vi "main_final.vi"() -> ()   [LabVIEW 2020]
uses:
  state.ctl
  <vilib>/MakerHub/LINX/Public/Utilities/Open Serial.vi
  <vilib>/MakerHub/LINX/Public/Sensors/Motion/Servo/Servo Open One Channel.vi
  <vilib>/MakerHub/LINX/Public/Sensors/Motion/Servo/Servo Close One Channel.vi
  <vilib>/MakerHub/LINX/LMH-LINX.lvlib
  <vilib>/MakerHub/LINX/Public/Sensors/Motion/Servo/Servo.lvlib
panel:
  in  "Buzzer":u8=12
  in  "Servo":u8=11
  in  "Serial Port":refnum<visa-resource-name>="N/A"
  out "message":string
  out "temp 2":dbl format="%#_3g"
  in  "temp":dbl(slide)=23.33965844402277 scale=0.0..100.0 scale format="%#_3g"
  out "Meter":dbl(knob) scale=1.0..5.0
  out "down":bool
  out "up":bool
  out "count":i32
  in  "hold":bool
  out "5":u16(ring)
  out "4":u16(ring)
  out "3":u16(ring)
  out "2":u16(ring)
  out "1":u16(ring)
  out "1":i8
  out "2":i8
  out "4":i8
  out "3":i8
  out "5":i8
  in  "up/down":T1
  in  "floor cluster":T2
  in  "Stop":bool
  out "floor":dbl(slide) scale=10.0..50.0
  # "Reset in :"
  # "Sec"
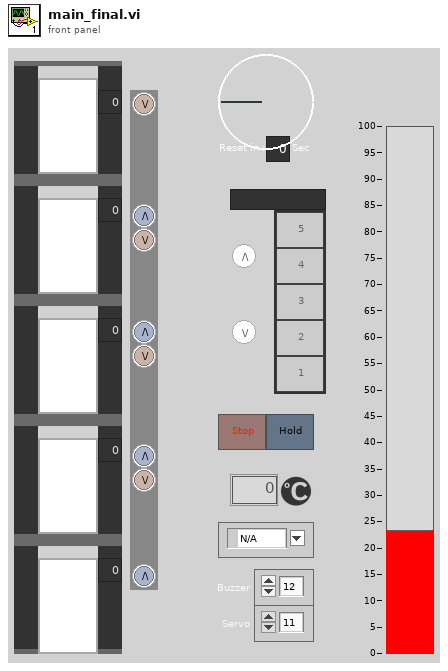
[diagram p1: front panel]
types:
  T1 = cluster{"up":bool, "down 2":bool, "up 2":bool, "down 3":bool, "up 3":bool, "down 4":bool, "up 4":bool, "down 5":bool}
  T2 = cluster{"1":bool, "2":bool, "3":bool, "4":bool, "5":bool}
  T3 = typedef "state.ctl" = enum16{"enter", "checking", "go up", "go down", "process", "get out", "temp"}
  T4 = typedef "LMH-LINX.lvlib/LINX Ref.ctl" = cluster{"IO":T5, "Interface":T6, "LINX Device Config":T7}
  T5 = typedef "LMH-LINX.lvlib/Platform.ctl" = enum16{"Remote", "Local"}
  T6 = typedef "LMH-LINX.lvlib/Interface.ctl" = enum16{"Serial", "TCP"}
  T7 = typedef "LMH-LINX.lvlib/Device.lvlib/LINX Device Config.ctl" = cluster{"Interface":T6, "COM Port":refnum<visa-resource-name>, "TCP Configuration":T8, "Device Family":u8, "Device ID":u8, "Device Name":string, "TCP Ref":refnum<k5>, "Channels":T9}
  T8 = typedef "LMH-LINX.lvlib/Device.lvlib/TCP Config.ctl" = cluster{"IP Address":string, "Port":u16}
  T9 = typedef "LMH-LINX.lvlib/Channels.ctl" = cluster{"DI":u8[], "DO":u8[], "AI":u8[], "AO":u8[], "PWM":u8[], "QE":u8[], "UART":u8[], "I2C 2":u8[], "SPI":u8[], "CAN":u8[], "Servo":u8[], "AI Ref (V)":dbl, "AI Resolution (Bits)":u8, "AO Ref (V)":dbl, "AO Resolution (Bits)":u8}
  T10 = enum8{"Enabled", "Disabled", "Disabled and Grayed Out"}
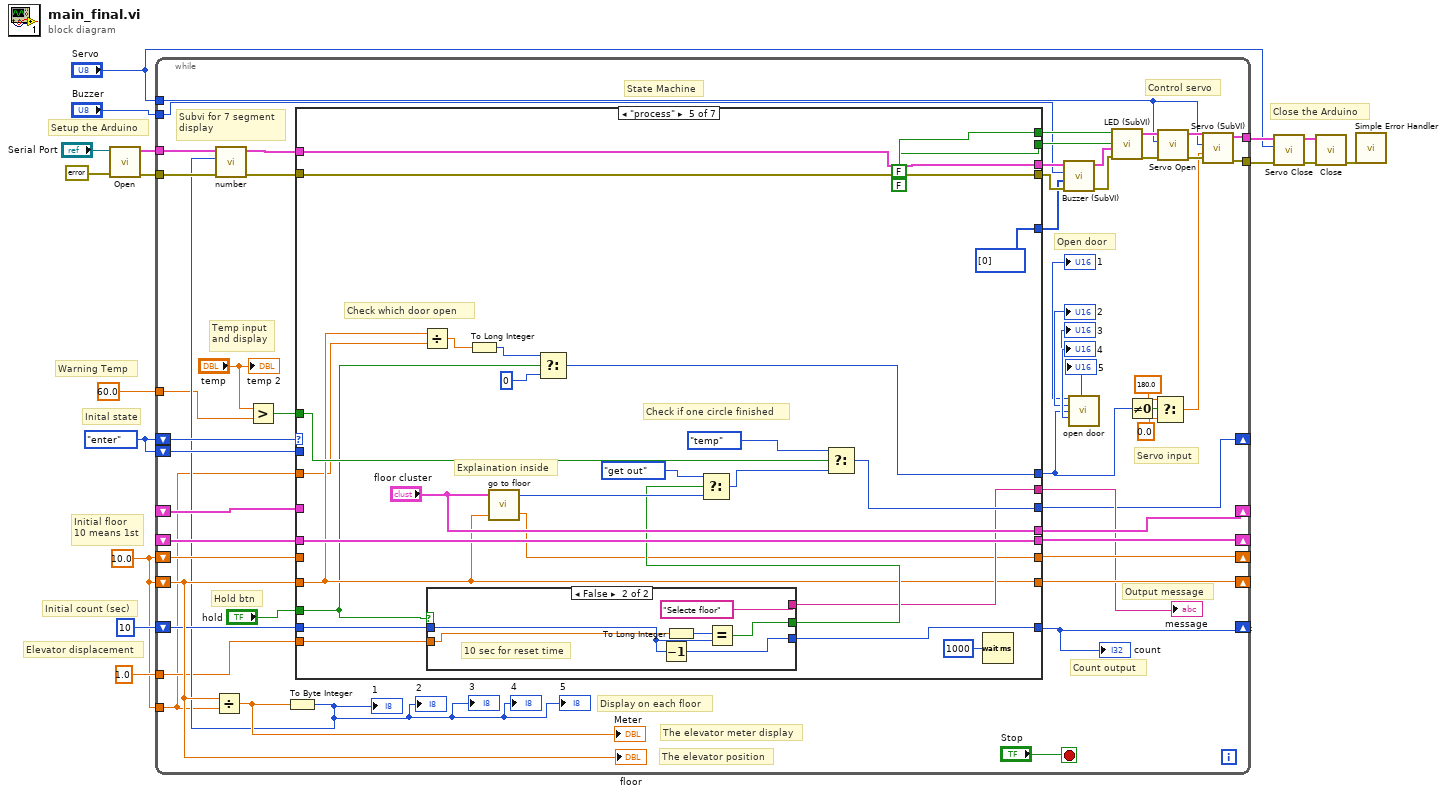
[diagram p0: block diagram]
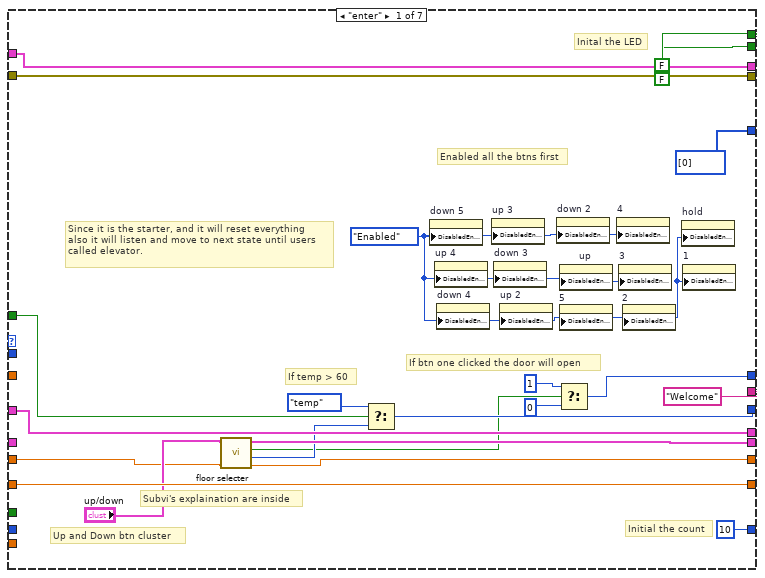
[diagram p2: hidden frame]
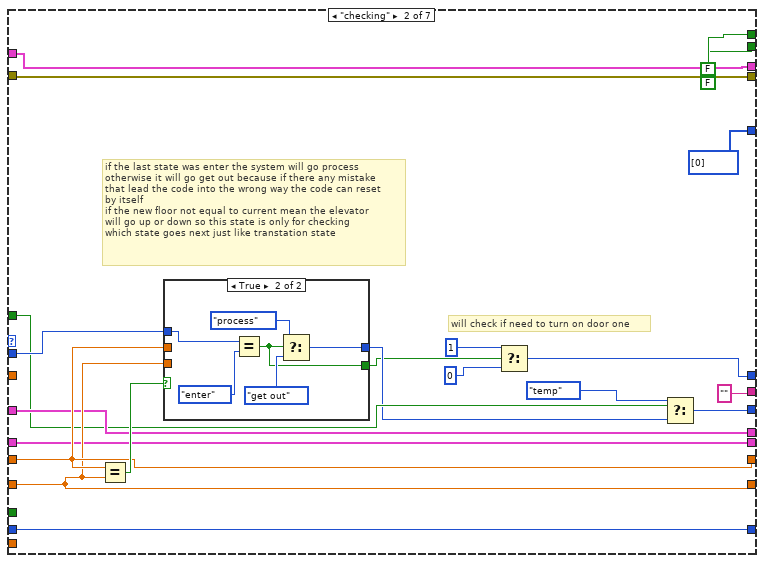
[diagram p3: hidden frame]
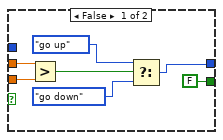
[diagram p4: hidden frame]
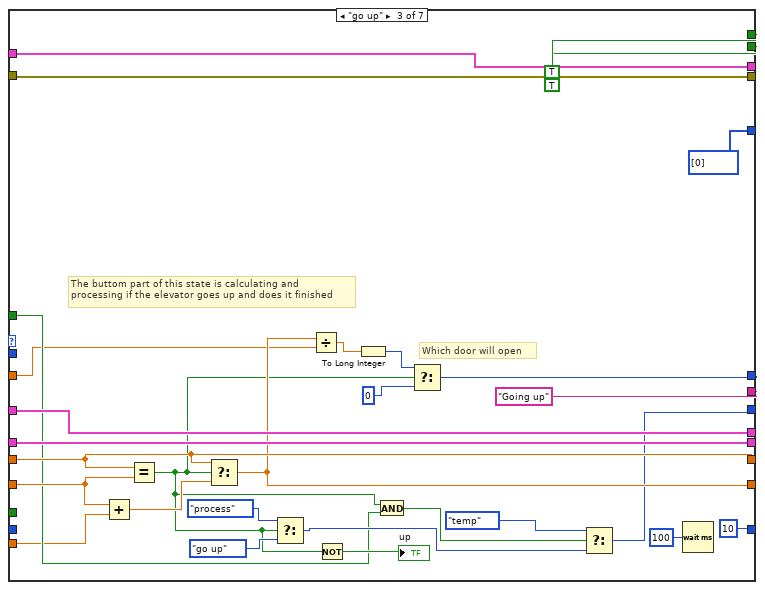
[diagram p5: hidden frame]
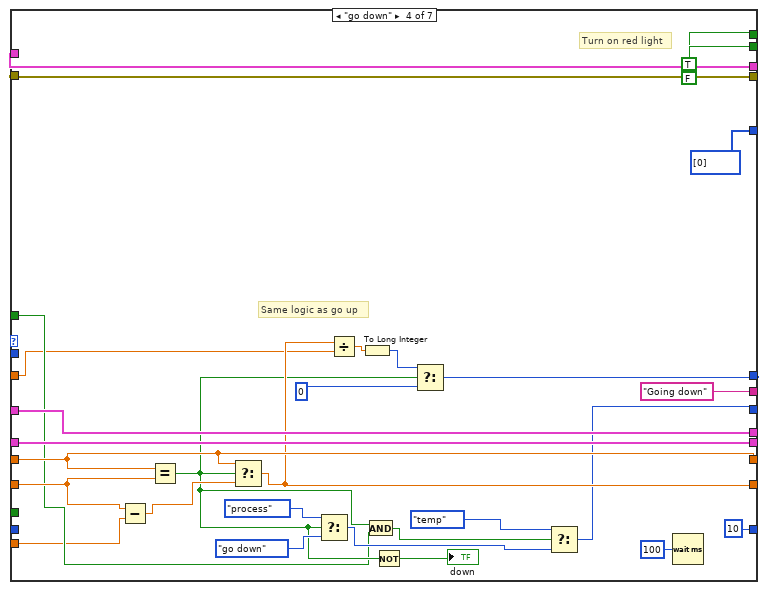
[diagram p6: hidden frame]
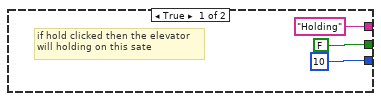
[diagram p7: hidden frame]
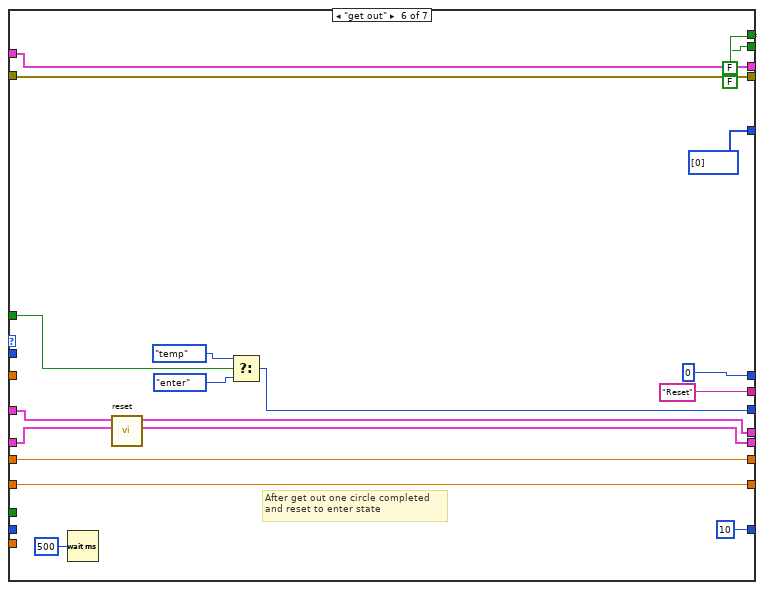
[diagram p8: hidden frame]
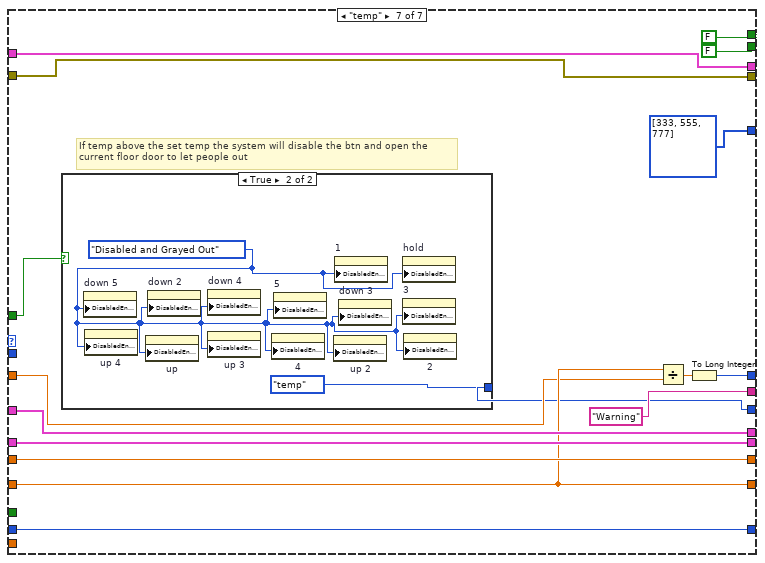
[diagram p9: hidden frame]
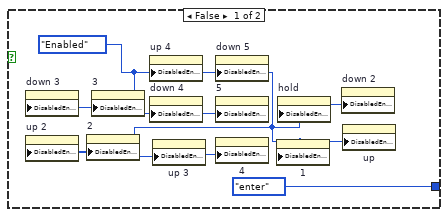
[diagram p10: hidden frame]
diagram:
  w3 = 10.0 ("floor")
  w15 = state."enter"
  # "Close the Arduino"
  # "Warning Temp"
  # "Elevator displacement"
  # "Initial count (sec)"
  # "Setup the Arduino"
  # "Initial floor\n10 means 1st"
  # "Inital state"
  n1 = call-poly <vilib>:"Open.vi"("Error In"=errorcluster {"status"=FALSE, "code"=0, "source"=""}, "Serial Port"="Serial Port") -> ("Error Out"=w10:errorcluster, "LINX Resource"=w11:T4)  [unwired: 7 in, 1 out]
  n2 = while {
    shift-right: [w26] -> _
    shift-left: w15 -> [w60]
    shift-right: [w66] -> _
    shift-left: w3 -> [w67]
    shift-right: [w59] -> _
    shift-left: _ -> [w65]
    shift-right: [w64] -> _
    shift-left: w3 -> [w63]
    shift-right: [w62] -> _
    shift-left: _ -> [w61]
    shift-right: [w31] -> _
    shift-left: 10 ("count") -> [w58]
    shift-left: w15 -> [w57]
    tunnel: w11 -> [w50]
    tunnel: w10 -> [w49]
    tunnel: [w47] -> w9
    tunnel: [w46] -> w8
    tunnel: "Servo" -> [w23]
    tunnel: 1.0 ("y") -> [w29]
    tunnel: w3 -> [w28]
    tunnel: 60.0 -> [w27]
    tunnel: "Buzzer" -> [w18]
    stop <- "Stop" stop-if-true
    # "Control servo"
    # "Servo input"
    # "Open door"
    # "State Machine"
    # "Output message"
    # "Count output"
    # "Display on each floor"
    # "The elevator meter display"
    # "The elevator position"
    # "Hold btn"
    # "Temp input\nand display"
    # "Subvi for 7 segment\ndisplay"
    n3 = Divide(x=w63, y=w28) -> (x/y=w51:dbl)
    "Meter" <- w51
    n4 = Greater?(x="temp", y=w27) -> (0:w55:bool)
    n5 = To Byte Integer(number=w51) -> (8bit integer=w41:i8)
    "5" <- w41
    "3" <- w41
    "4" <- w41
    "2" <- w41
    "1" <- w41
    n6 = call "number.vi"("error in (no error)"=w49, "Numeric"=w41, "LINX Resource in"=w50) -> ("error out"=w24:errorcluster, "LINX Resource out"=w48:T4)  [unwired: 7 in]
    n7 = case shown="\"process\"" w60 {
      tunnel: w67 -> [w78 w110 w152 w179 _ w237 w251]
      tunnel: [w76 w108 w153 w182 w208 w221 w252] -> w59
      tunnel: [w77 w110 w152 w179 w185 w237 w251] -> w66
      tunnel: w65 -> [_ w108 w153 w182 w208 w220 w252]
      tunnel: [w86 w101 w137 w166 w196 w228 w239] -> w26
      tunnel: [w90 w109 w142 w171 w189 w235 w247] -> w64
      tunnel: w63 -> [w90 w109 w149 w177 w189 w235 w247]
      tunnel: [w89 w107 w146 w175 "floor cluster" w222 w253] -> w62
      tunnel: w61 -> [w89 w107 w146 w175 _ w234 w253]
      tunnel: [w71 w94 w143 w173 w203 0 ("f") w248] -> w32
      tunnel: [10 w105 10 ("count") 10 ("count") w207 10 w250] -> w31
      tunnel: w58 -> [_ w105 _ _ w200 _ w250]
      tunnel: w57 -> [_ w106 _ _ _ _ _]
      tunnel: "hold" -> [_ _ _ _ w188 _ _]
      tunnel: w55 -> [w85 w103 w135 w164 w197 w229 w240]
      tunnel: ["Welcome" "" "Going up" "Going down" w190 "Reset" "Warning"] -> w54
      tunnel: w29 -> [_ _ w131 w161 w186 _ _]
      tunnel: w48 -> [w70 w93 w128 w158 w184 w223 w243]
      tunnel: w24 -> [w81 w98 w127 w157 w192 w224 w241]
      tunnel: [FALSE ("On/OFF") FALSE ("On/OFF") TRUE ("On/OFF") TRUE ("On/OFF") FALSE ("On/OFF") FALSE ("On/OFF") FALSE ("On/OFF")] -> w53
      tunnel: [FALSE ("Blue / Red") FALSE ("Blue / Red") TRUE ("Blue / Red") FALSE ("Blue / Red") FALSE ("Blue / Red") FALSE ("Blue / Red") FALSE ("Blue / Red")] -> w52
      tunnel: [w70 w93 w128 w158 w184 w223 w243] -> w20
      tunnel: [w81 w98 w127 w157 w192 w224 w241] -> w19
      tunnel: w28 -> [_ _ w126 w156 w187 _ w242]
      tunnel: [i32[] [0] ("Array") i32[] [0] ("Array") i32[] [0] ("Array") i32[] [0] ("Array") i32[] [0] ("Array") i32[] [0] ("Array") i32[] [333, 555, 777] ("Array")] -> w17
      frame "enter" {
        w80 = T10."Enabled" ("Disabled")
        # "If btn one clicked the door will open"
        # "Subvi's explaination are inside"
        # "Since it is the starter, and it will reset everything\nalso it will listen and move to next state until users\ncalled elevator."
        # "If temp > 60"
        # "Initial the count"
        # "Inital the LED"
        # "Enabled all the btns first"
        # "Up and Down btn cluster"
        n8 = call "floor selecter.vi"("floor in"=w78, "up/down in"="up/down") -> ("floor out"=w77:dbl, "state"=w75:T3, "T/F"=w74:bool, "up/down out"=w76:T1)  [unwired: 3 in]
        n9 = Select(t=state."temp", s=w85, f=w75) -> (s? t:f=w86:T3)
        n10 = property on="down 5" class="Bool"("DisabledEnum"=w80) -> ()  [unwired: 2 in, 2 out]
        n11 = property on="up 4" class="Bool"("DisabledEnum"=w80) -> ()  [unwired: 2 in, 2 out]
        n12 = property on="down 4" class="Bool"("DisabledEnum"=w80) -> ()  [unwired: 2 in, 2 out]
        n13 = property on="up 3" class="Bool"("DisabledEnum"=w80) -> ()  [unwired: 2 in, 2 out]
        n14 = property on="down 3" class="Bool"("DisabledEnum"=w80) -> ()  [unwired: 2 in, 2 out]
        n15 = property on="up 2" class="Bool"("DisabledEnum"=w80) -> ()  [unwired: 2 in, 2 out]
        n16 = property on="down 2" class="Bool"("DisabledEnum"=w80) -> ()  [unwired: 2 in, 2 out]
        n17 = Select(t=1 ("f"), s=w74, f=0) -> (s? t:f=w71:i32)
        n18 = property on="up" class="Bool"("DisabledEnum"=w80) -> ()  [unwired: 2 in, 2 out]
        n19 = property on="5" class="Bool"("DisabledEnum"=w80) -> ()  [unwired: 2 in, 2 out]
        n20 = property on="4" class="Bool"("DisabledEnum"=w80) -> ()  [unwired: 2 in, 2 out]
        n21 = property on="3" class="Bool"("DisabledEnum"=w80) -> ()  [unwired: 2 in, 2 out]
        n22 = property on="2" class="Bool"("DisabledEnum"=w80) -> ()  [unwired: 2 in, 2 out]
        n23 = property on="hold" class="Bool (strict)"("DisabledEnum"=w80) -> ()  [unwired: 2 in, 2 out]
        n24 = property on="1" class="Bool"("DisabledEnum"=w80) -> ()  [unwired: 2 in, 2 out]
      }
      frame "checking" {
        # "will check if need to turn on door one"
        # "if the last state was enter the system will go process\notherwise it will go get out because if there any mistake\nthat lead the code into the wrong way the code can reset\nby itself\nif the new floor not equal to current mean the elevator\nwill go up or down so this state is only for checking\nwhich state goes next just like transtation state"
        n25 = Equal?(x=w110, y=w109) -> (x = y?=w111:bool)
        n26 = case shown="True" w111 {
          tunnel: w110 -> [w118 _]
          tunnel: w109 -> [w117 _]
          tunnel: [w113 w120] -> w102
          tunnel: w106 -> [_ w124]
          tunnel: [FALSE w119] -> w97
          frame False {
            n27 = Greater?(x=w118, y=w117) -> (0:w116:bool)
            n28 = Select(t=state."go up", s=w116, f=state."go down") -> (s? t:f=w113:T3)
          }
          frame True {
            n29 = Equal?(x=w124, y=state."enter") -> (x = y?=w119:bool)
            n30 = Select(t=state."process", s=w119, f=state."get out") -> (s? t:f=w120:T3)
          }
        }
        n31 = Select(t=1 ("f"), s=w97, f=0) -> (s? t:f=w94:i32)
        n32 = Select(t=state."temp", s=w103, f=w102) -> (s? t:f=w101:T3)
      }
      frame "go up" {
        # "The buttom part of this state is calculating and\nprocessing if the elevator goes up and does it finished"
        # "Which door will open"
        n33 = Add(x=w149, y=w131) -> (x+y=w148:dbl)
        n34 = Equal?(x=w152, y=w149) -> (x = y?=w136:bool)
        n35 = Select(t=w152, s=w136, f=w148) -> (s? t:f=w142:dbl)
        n36 = Select(t=state."process", s=w136, f=state."go up") -> (s? t:f=w138:T3)
        n37 = Divide(x=w142, y=w126) -> (x/y=w141:dbl)
        n38 = Not(x=w136) -> (.not. x?=→"up":bool)
        n39 = To Long Integer(number=w141) -> (32bit integer=w144:i32)
        n40 = And(x=w136, y=w135) -> (x .and. y?=w134:bool)
        n41 = Select(t=w144, s=w136, f=0) -> (s? t:f=w143:i32)
        n42 = Select(t=state."temp", s=w134, f=w138) -> (s? t:f=w137:T3)
        n43 = Wait (ms)(milliseconds to wait=u32 100) -> ()  [unwired: 1 out]
      }
      frame "go down" {
        # "Turn on red light"
        # "Same logic as go up"
        n44 = Subtract(x=w177, y=w161) -> (x-y=w176:dbl)
        n45 = Equal?(x=w179, y=w177) -> (x = y?=w165:bool)
        n46 = Select(t=w179, s=w165, f=w176) -> (s? t:f=w171:dbl)
        n47 = Select(t=state."process", s=w165, f=state."go down") -> (s? t:f=w167:T3)
        n48 = Divide(x=w171, y=w156) -> (x/y=w170:dbl)
        n49 = To Long Integer(number=w170) -> (32bit integer=w172:i32)
        n50 = And(x=w165, y=w164) -> (x .and. y?=w163:bool)
        n51 = Not(x=w165) -> (.not. x?=→"down":bool)
        n52 = Select(t=w172, s=w165, f=0) -> (s? t:f=w173:i32)
        n53 = Select(t=state."temp", s=w163, f=w167) -> (s? t:f=w166:T3)
        n54 = Wait (ms)(milliseconds to wait=u32 100) -> ()  [unwired: 1 out]
      }
      frame "process" {
        # "Check if one circle finished"
        # "Explaination inside"
        # "Check which door open"
        n55 = Divide(x=w189, y=w187) -> (x/y=w204:dbl)
        n56 = case shown="False" w188 {
          tunnel: [10 w218] -> w207
          tunnel: w200 -> [_ w217]
          tunnel: [FALSE w216] -> w191
          tunnel: ["Holding" "Selecte floor"] -> w190
          tunnel: w186 -> [_ w214]
          frame True {
            # "if hold clicked then the elevator\nwill holding on this sate"
          }
          frame False {
            # "10 sec for reset time"
            n57 = Decrement(x=w217) -> (x-1=w218:i32)
            n58 = To Long Integer(number=w214) -> (32bit integer=w213:i32)
            n59 = Equal?(x=w213, y=w217) -> (x = y?=w216:bool)
          }
        }
        n60 = To Long Integer(number=w204) -> (32bit integer=w202:i32)
        n61 = call "go to floor.vi"("current floor in"=w189, "floor cluster in"="floor cluster") -> ("new floor out"=w185:dbl, "state out"=w206:T3)  [unwired: 1 in]
        n62 = Select(t=w202, s=w188, f=0) -> (s? t:f=w203:i32)
        n63 = Select(t=state."get out", s=w191, f=w206) -> (s? t:f=w198:T3)
        n64 = Select(t=state."temp", s=w197, f=w198) -> (s? t:f=w196:T3)
        n65 = Wait (ms)(milliseconds to wait=u32 1000) -> ()  [unwired: 1 out]
      }
      frame "get out" {
        # "After get out one circle completed\nand reset to enter state"
        n66 = Wait (ms)(milliseconds to wait=u32 500) -> ()  [unwired: 1 out]
        n67 = call "reset.vi"("up/down in"=w220, "floor cluster in"=w234) -> ("up/down out"=w221:T1, "floor cluster out"=w222:T2)  [unwired: 8 in]
        n68 = Select(t=state."temp", s=w229, f=state."enter") -> (s? t:f=w228:T3)
      }
      frame "temp" {
        # "If temp above the set temp the system will disable the btn and open the\ncurrent floor door to let people out"
        n69 = case shown="True" w240 {
          tunnel: [state."enter" state."temp"] -> w239
          frame False {
            w254 = T10."Enabled" ("Disabled")
            n70 = property on="down 3" class="Bool"("DisabledEnum"=w254) -> ()  [unwired: 2 in, 2 out]
            n71 = property on="up 2" class="Bool"("DisabledEnum"=w254) -> ()  [unwired: 2 in, 2 out]
            n72 = property on="2" class="Bool"("DisabledEnum"=w254) -> ()  [unwired: 2 in, 2 out]
            n73 = property on="3" class="Bool"("DisabledEnum"=w254) -> ()  [unwired: 2 in, 2 out]
            n74 = property on="up 4" class="Bool"("DisabledEnum"=w254) -> ()  [unwired: 2 in, 2 out]
            n75 = property on="down 4" class="Bool"("DisabledEnum"=w254) -> ()  [unwired: 2 in, 2 out]
            n76 = property on="up 3" class="Bool"("DisabledEnum"=w254) -> ()  [unwired: 2 in, 2 out]
            n77 = property on="down 5" class="Bool"("DisabledEnum"=w254) -> ()  [unwired: 2 in, 2 out]
            n78 = property on="5" class="Bool"("DisabledEnum"=w254) -> ()  [unwired: 2 in, 2 out]
            n79 = property on="4" class="Bool"("DisabledEnum"=w254) -> ()  [unwired: 2 in, 2 out]
            n80 = property on="1" class="Bool"("DisabledEnum"=w254) -> ()  [unwired: 2 in, 2 out]
            n81 = property on="hold" class="Bool (strict)"("DisabledEnum"=w254) -> ()  [unwired: 2 in, 2 out]
            n82 = property on="down 2" class="Bool"("DisabledEnum"=w254) -> ()  [unwired: 2 in, 2 out]
            n83 = property on="up" class="Bool"("DisabledEnum"=w254) -> ()  [unwired: 2 in, 2 out]
          }
          frame True {
            w256 = T10."Disabled and Grayed Out" ("Disabled")
            n84 = property on="down 5" class="Bool"("DisabledEnum"=w256) -> ()  [unwired: 2 in, 2 out]
            n85 = property on="up 4" class="Bool"("DisabledEnum"=w256) -> ()  [unwired: 2 in, 2 out]
            n86 = property on="up" class="Bool"("DisabledEnum"=w256) -> ()  [unwired: 2 in, 2 out]
            n87 = property on="down 2" class="Bool"("DisabledEnum"=w256) -> ()  [unwired: 2 in, 2 out]
            n88 = property on="down 4" class="Bool"("DisabledEnum"=w256) -> ()  [unwired: 2 in, 2 out]
            n89 = property on="up 3" class="Bool"("DisabledEnum"=w256) -> ()  [unwired: 2 in, 2 out]
            n90 = property on="4" class="Bool"("DisabledEnum"=w256) -> ()  [unwired: 2 in, 2 out]
            n91 = property on="5" class="Bool"("DisabledEnum"=w256) -> ()  [unwired: 2 in, 2 out]
            n92 = property on="up 2" class="Bool"("DisabledEnum"=w256) -> ()  [unwired: 2 in, 2 out]
            n93 = property on="1" class="Bool"("DisabledEnum"=w256) -> ()  [unwired: 2 in, 2 out]
            n94 = property on="down 3" class="Bool"("DisabledEnum"=w256) -> ()  [unwired: 2 in, 2 out]
            n95 = property on="hold" class="Bool (strict)"("DisabledEnum"=w256) -> ()  [unwired: 2 in, 2 out]
            n96 = property on="3" class="Bool"("DisabledEnum"=w256) -> ()  [unwired: 2 in, 2 out]
            n97 = property on="2" class="Bool"("DisabledEnum"=w256) -> ()  [unwired: 2 in, 2 out]
          }
        }
        n98 = Divide(x=w247, y=w242) -> (x/y=w249:dbl)
        n99 = To Long Integer(number=w249) -> (32bit integer=w248:i32)
      }
    }
    "message" <- w54
    "count" <- w31
    n100 = call "Buzzer (SubVI).vi"("error in (no error)"=w19, "Array"=w17, "Digital Pin"=w18, "LINX Resource in"=w20) -> ("error out"=w21:errorcluster, "LINX Resource out"=w22:T4)  [unwired: 6 in]
    n101 = call "open door.vi"("input"=w32) -> ("1"=→"1":u16, "2"=→"2":u16, "3"=→"3":u16, "4"=→"4":u16, "5"=→"5":u16)  [unwired: 10 in]
    n102 = call "LED (SubVI).vi"("error in (no error)"=w21, "LINX Resource in"=w22, "Blue / Red"=w52, "On/OFF"=w53) -> ("error out"=w44:errorcluster, "LINX Resource out"=w45:T4)
    n103 = Not Equal To 0?(x=w32) -> (x != 0?=w30:bool)
    n104 = Select(t=180.0, s=w30, f=0.0) -> (s? t:f=w33:dbl)
    n105 = call-poly <vilib>:"Servo Open.vi"("Error In"=w44, "Servo Channel"=w23, "LINX Resource"=w45) -> ("Error Out"=w42:errorcluster, "LINX Resource"=w43:T4)  [unwired: 7 in]
    n106 = call "Servo (SubVI).vi"("error in (no error)"=w42, "Position in"=w33, "Servo Channel"=w23, "LINX Resource in"=w43) -> ("error out"=w46:errorcluster, "LINX Resource out"=w47:T4)  [unwired: 5 in, 1 out]
    "floor" <- w63
    "temp 2" <- "temp"
  }
  n107 = call-poly <vilib>:"Servo Close.vi"("Error In"=w8, "Servo Channel"="Servo", "LINX Resource"=w9) -> ("Error Out"=w6:errorcluster, "LINX Resource"=w7:T4)  [unwired: 7 in]
  n108 = call <vilib>:"Close.vi"("Error In"=w6, "LINX Resource"=w7) -> ("Error Out"=w12:errorcluster)  [unwired: 9 in]
  n109 = call <vilib>:"Simple Error Handler.vi"("error in (no error)"=w12) -> ()  [unwired: 4 in, 5 out]
